vi "Axes to mspec stitcher calib cluster.vi"(10 "Angle axis":dbl[](array[numeric]), 11 "Energy axis":dbl[](array[numeric])) -> (3 "calib":T1)   [LabVIEW 2013, in "MagSpecStitcher.lvclass"]
uses:
  MagSpecStitcher.lvclass
  LineoutStats.ctl
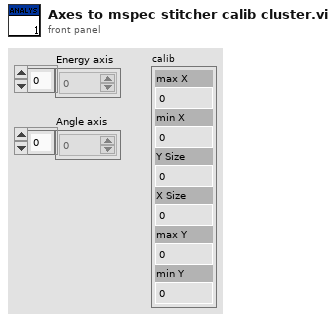
[diagram p1: front panel]
types:
  T1 = typedef "LineoutStats.ctl" = cluster{"max X":dbl, "min X":dbl, "Y Size":dbl, "X Size":dbl, "max Y":dbl, "min Y":dbl}
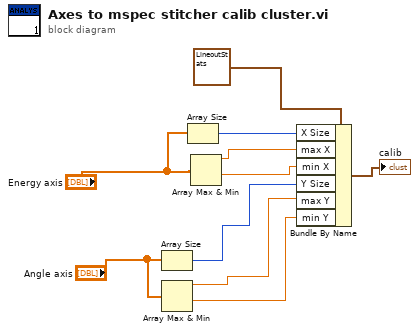
[diagram p0: block diagram]
diagram:
  n1 = Array Size(array="Angle axis") -> (size(s)=w4:i32)
  n2 = Array Max & Min(array="Angle axis") -> (max value=w9:dbl, min value=w10:dbl)  [unwired: 2 out]
  n3 = Array Size(array="Energy axis") -> (size(s)=w8:i32)
  n4 = Array Max & Min(array="Energy axis") -> (max value=w1:dbl, min value=w2:dbl)  [unwired: 2 out]
  n5 = Bundle By Name(cluster=T1 {"max X"=71.374177, "min X"=34.374177, "Y Size"=95.0, "X Size"=95.0, "max Y"=0.0, "min Y"=0.0} ("calib"), "X Size"=w8, "max X"=w1, "min X"=w2, "Y Size"=w4, "max Y"=w9, "min Y"=w10) -> (→"calib":T1)
